vi "SubtractionUI.vi"(0 "Subtract in":refnum<class "Subtract.lvclass">, 1 "B":dbl, 5 "A":dbl, 7 "user event out":refnum<user-event>, 9 "event source":refnum<user-event>, 11 "error in (no error)":errorcluster, 12 "Calculate":bool) -> (4 "Subtract out":refnum<class "Subtract.lvclass">, 6 "C":dbl, 15 "error out":errorcluster)   [LabVIEW 2023, in "Subtract.lvclass"]
uses:
  Subtract.lvclass
  C:/Users/santharu.subramanian/Documents/LV New Assignments/DVR in OOPS/Classes/Arithmetic/Arithmetic.lvclass
  Arithmetic/Arithmetic.lvclass
  Subtract.lvclass/Subtract.ctl
panel:
  # "SUBTRACTION"
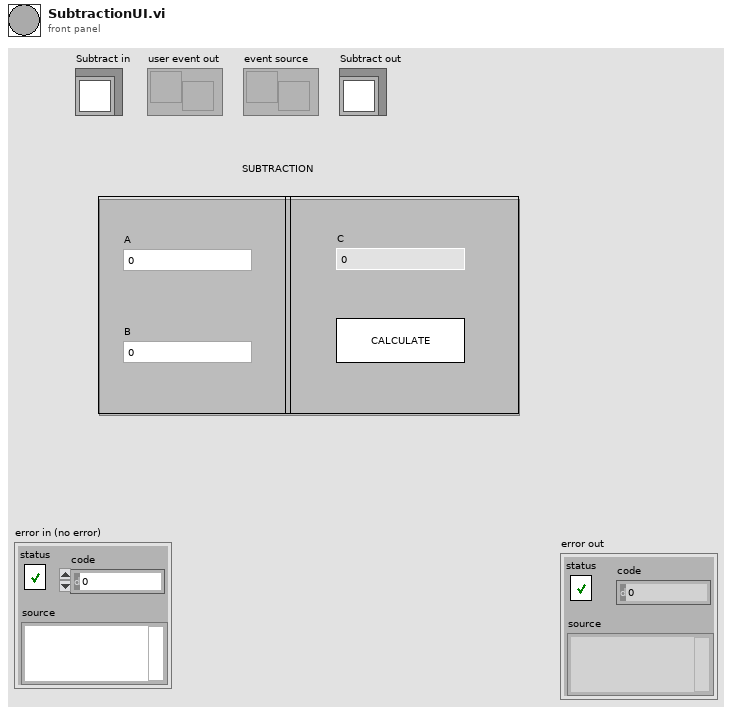
[diagram p1: front panel]
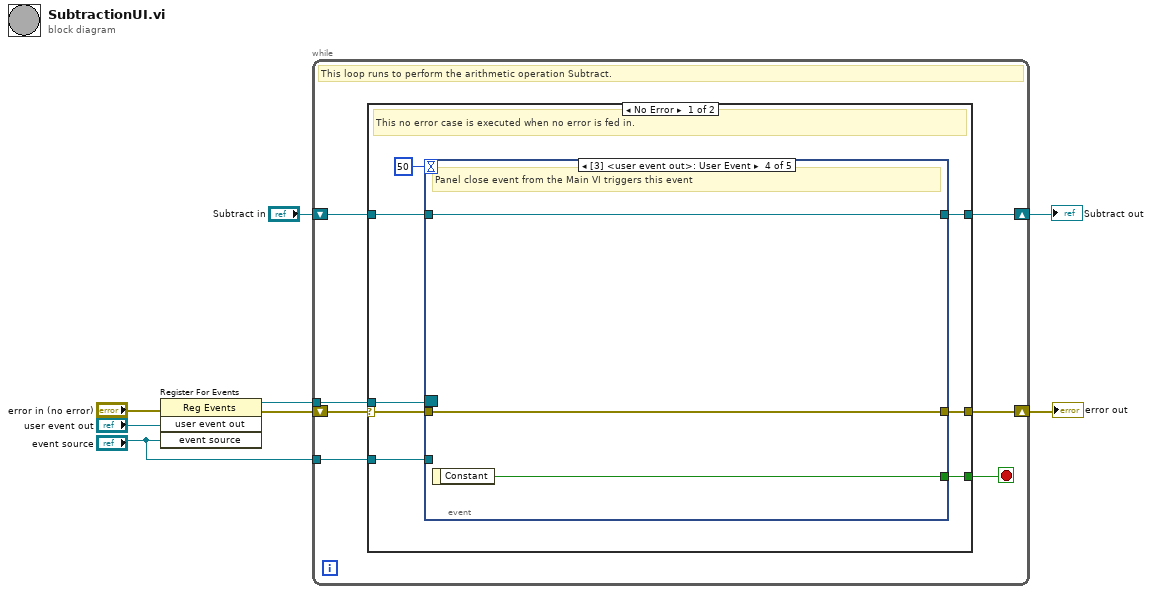
[diagram p0: block diagram]
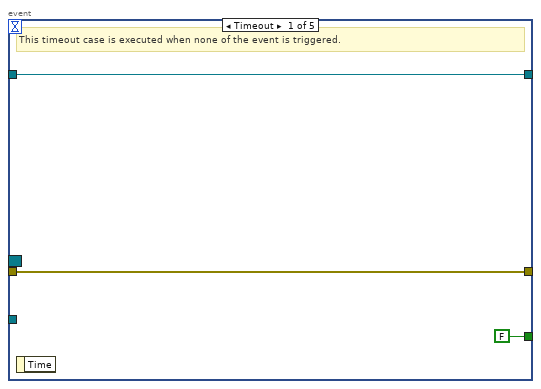
[diagram p2: hidden frame]
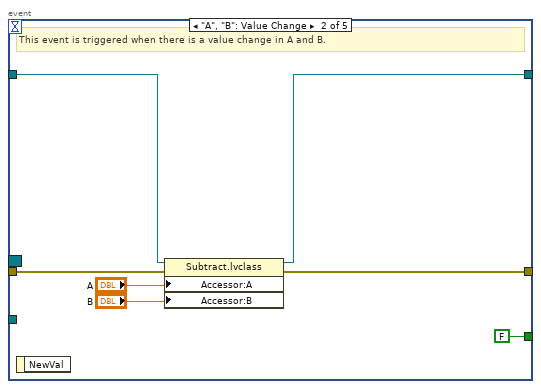
[diagram p3: hidden frame]
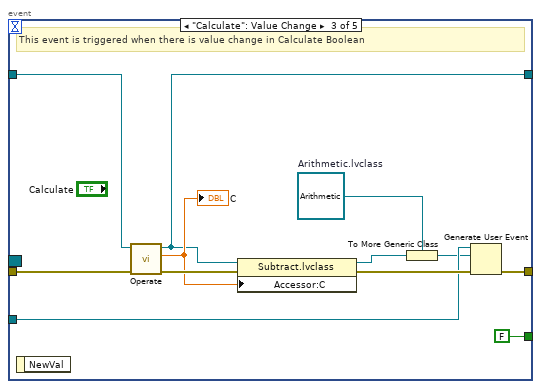
[diagram p4: hidden frame]
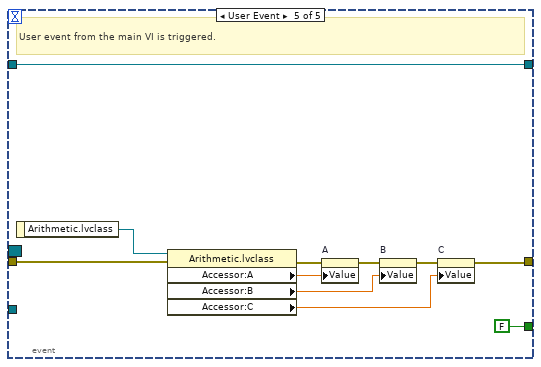
[diagram p5: hidden frame]
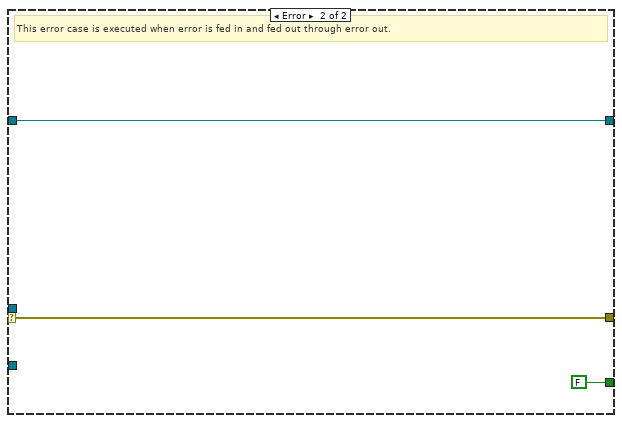
[diagram p6: hidden frame]
diagram:
  n1 = register-events(error in="error in (no error)", "user event out", "event source") -> (reference out=w2:refnum<event-registration>, error out=w3:errorcluster)  [unwired: 1 in]
  n2 = while {
    shift-right: [w14] -> w6
    shift-left: w3 -> [w15]
    shift-right: [w12] -> w7
    shift-left: "Subtract in" -> [w13]
    tunnel: w2 -> [w11]
    tunnel: "event source" -> [w9]
    stop <- w10 stop-if-true
    # "This loop runs to perform the arithmetic operation Subtract."
    n3 = case shown="No Error" w15 {
      selector: w15 -> [w23 w62]
      tunnel: [w22 w62] -> w14
      tunnel: [w20 w61] -> w12
      tunnel: w13 -> [w21 w61]
      tunnel: w11 -> [w18 _]
      tunnel: [w17 FALSE ("Constant")] -> w10
      tunnel: w9 -> [w16 _]
      frame No Error {
        # "This no error case is executed when no error is fed in."
        n4 = event shown="[3] <user event out>: User Event" {
          selector: w18 -> [_ _ _ _ _]
          dyn-events: _ -> [_ _ _ _ _]
          timeout: 50 -> [_ _ _ _ _]
          tunnel: w23 -> [w26 w32 w44 w47 w50]
          tunnel: [w26 w31 w40 w47 w49] -> w22
          tunnel: w21 -> [w25 w33 w45 w48 w59]
          tunnel: [w25 w28 w38 w48 w59] -> w20
          tunnel: [FALSE ("Constant") FALSE ("Constant") FALSE ("Constant") w46 FALSE ("Constant")] -> w17
          tunnel: w16 -> [_ _ w37 _ _]
          event Timeout {
            # "This timeout case is executed when none of the event is triggered."
            n5 = event-data() -> ()  [unwired: 1 in, 1 out]
          }
          event "A", "B": Value Change {
            # "This event is triggered when there is a value change in A and B."
            n6 = event-data() -> ()  [unwired: 1 in, 1 out]
            n7 = property class="Subtract.lvclass"(reference=w33, error in=w32, "Accessor:A"="A", "Accessor:B"="B") -> (reference out=w28:refnum<class "Subtract.lvclass">, error out=w31:errorcluster)
          }
          event "Calculate": Value Change {
            w34 = refnum<class "Arithmetic.lvclass"> refnum  # Arithmetic.lvclass
            # "This event is triggered when there is value change in Calculate Boolean"
            n8 = event-data() -> ()  [unwired: 1 in, 1 out]
            n9 = call-dynamic "Operate.vi"("error in (no error)"=w44, "Subtract in"=w45) -> ("error out"=w41:errorcluster, "C"=w39:dbl, "Subtract out"=w38:refnum<class "Subtract.lvclass">)  [unwired: 7 in]
            "C" <- w39
            n10 = property class="Subtract.lvclass"(reference=w38, error in=w41, "Accessor:C"=w39) -> (reference out=w42:refnum<class "Subtract.lvclass">, error out=w43:errorcluster)
            n11 = To More Generic Class(target class=w34, reference=w42) -> (generic class reference=w35:refnum<class "Arithmetic.lvclass">)
            n12 = Generate User Event(user event=w37, event data cluster=w35, error in=w43) -> (error out=w40:errorcluster)  [unwired: 1 in, 1 out]
          }
          event User Event {
            # "Panel close event from the Main VI triggers this event"
            n13 = event-data() -> ("Constant"=w46:bool)  [unwired: 1 in]
          }
          event User Event {
            # "User event from the main VI is triggered."
            n14 = event-data() -> ("Arithmetic.lvclass"=w51:refnum<class "Arithmetic.lvclass">)  [unwired: 1 in]
            n15 = property class="Arithmetic.lvclass"(reference=w51, error in=w50) -> (error out=w57:errorcluster, "Accessor:A"=w56:dbl, "Accessor:B"=w53:dbl, "Accessor:C"=w52:dbl)  [unwired: 1 out]
            n16 = property on="A" class="DigNum (strict)"(error in=w57, "Value"=w56) -> (error out=w55:errorcluster)  [unwired: 1 in, 1 out]
            n17 = property on="B" class="DigNum (strict)"(error in=w55, "Value"=w53) -> (error out=w54:errorcluster)  [unwired: 1 in, 1 out]
            n18 = property on="C" class="DigNum (strict)"(error in=w54, "Value"=w52) -> (error out=w49:errorcluster)  [unwired: 1 in, 1 out]
          }
        }
      }
      frame Error {
        # "This error case is executed when error is fed in and fed out through error out."
      }
    }
  }
  "error out" <- w6
  "Subtract out" <- w7
